vi "Send Command.vi"(7 "Config offset":u64 format="%x", 8 "error in (no error)":errorcluster, 9 "Command payload":u64 format="%x", 10 "Command number":T1, 11 "RP Communicator in":refnum<class "RP Communicator VISA.lvclass">) -> (0 "error out":errorcluster, 3 "RP Communicator out":refnum<class "RP Communicator VISA.lvclass">)   [LabVIEW 2016, in "RP Communicator VISA.lvclass"]
uses:
  RP Communicator VISA.lvclass
  RP Command.ctl
  RP Write Command VISA.vi
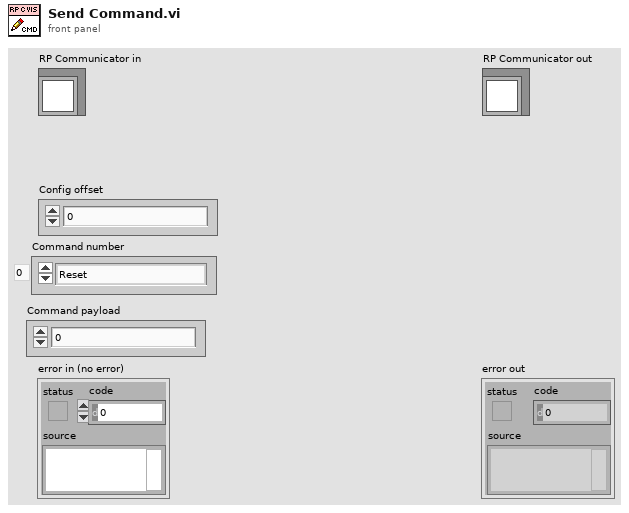
[diagram p1: front panel]
types:
  T1 = typedef "RP Command.ctl" = enum16{"Reset", "Read IDN", "Stop server", "Get status", "Get temperature", "Connect client", "Arm", "Software trigger", "Get whole buffer", "Get chunk", "System call", "Get config", "Set config", "Recieve data", "Play pattern", "Transmit data"}
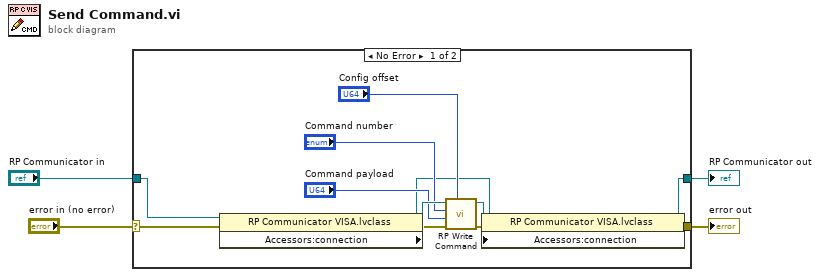
[diagram p0: block diagram]
diagram:
  n1 = case shown="No Error" "error in (no error)" {
    selector: "error in (no error)" -> [w8 w18]
    tunnel: [w5 w18] -> w3
    tunnel: [w10 w17] -> w1
    tunnel: "RP Communicator in" -> [w12 w17]
    frame No Error {
      n2 = property class="RP Communicator VISA.lvclass"(reference=w12, error in=w8) -> (reference out=w11:refnum<class "RP Communicator VISA.lvclass">, error out=w7:errorcluster, "Accessors:connection"=w16:refnum<visa-resource-name>)
      n3 = call-poly "RP Write Command.vi"("Config offset"="Config offset", "Error In"=w7, "Command payload"="Command payload", "Command number"="Command number", "VISA resource"=w16) -> ("Error Out"=w6:errorcluster, "VISA resource out"=w9:refnum<visa-resource-name>)  [unwired: 4 in, 1 out]
      n4 = property class="RP Communicator VISA.lvclass"(reference=w11, error in=w6, "Accessors:connection"=w9) -> (reference out=w10:refnum<class "RP Communicator VISA.lvclass">, error out=w5:errorcluster)
    }
    frame Error {
    }
  }
  "error out" <- w3
  "RP Communicator out" <- w1
